vi "Read String 1.vi"(8 "error in (no error)":errorcluster, 11 "Section 2 in":refnum<class "Section 2.lvclass">) -> (0 "error out":errorcluster, 2 "String 1":string="myString", 3 "Section 2 out":refnum<class "Section 2.lvclass">)   [LabVIEW 2015, in "LVOOP Introduction.lvlib" / "Section 2.lvclass"]
uses:
  Section 2.lvclass
  Section 2.lvclass/Section 2.ctl
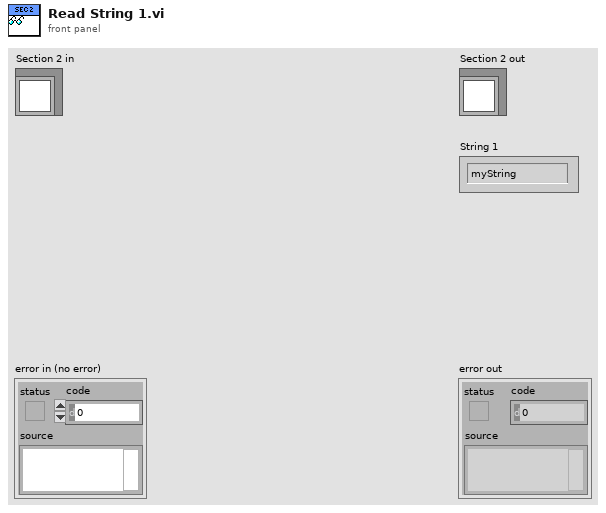
[diagram p1: front panel]
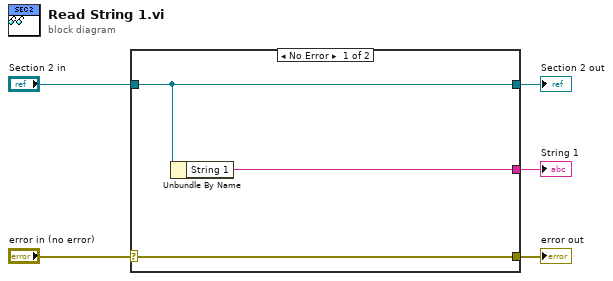
[diagram p0: block diagram]
diagram:
  n1 = case shown="No Error" "error in (no error)" {
    selector: "error in (no error)" -> [w8 w9]
    tunnel: [w8 w9] -> w4
    tunnel: [w7 w10] -> w2
    tunnel: "Section 2 in" -> [w7 w10]
    tunnel: [w6 _] -> w1
    frame No Error {
      n2 = Unbundle By Name(w7) -> ("String 1"=w6:string)
    }
    frame Error {
    }
  }
  "error out" <- w4
  "Section 2 out" <- w2
  "String 1" <- w1
